vi "Multistate LED Example LV2012.vi"() -> ()   [LabVIEW 2012]
panel:
  in  "stop":bool
  out "Color Box":u32(colorbox)
  in  "Enum":T1(ring)
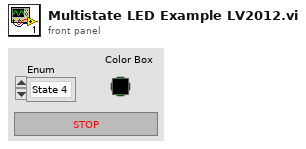
[diagram p1: front panel]
types:
  T1 = enum16{"State 4", "State 3", "State 2", "State 1", "State 0"}
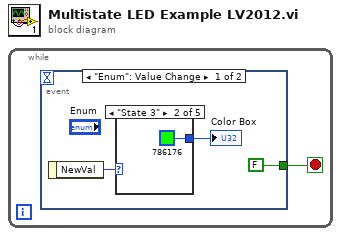
[diagram p0: block diagram]
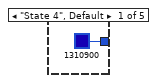
[diagram p2: hidden frame]
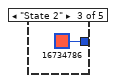
[diagram p3: hidden frame]
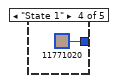
[diagram p4: hidden frame]
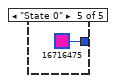
[diagram p5: hidden frame]
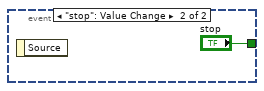
[diagram p6: hidden frame]
diagram:
  n1 = while {
    stop <- w1 stop-if-true
    n2 = event shown="[0] \"Enum\": Value Change" {
      selector: _ -> [_ _]
      dyn-events: _ -> [_ _]
      timeout: _ -> [_ _]
      tunnel: [FALSE ("stop") "stop"] -> w1
      event "Enum": Value Change {
        n3 = event-data() -> ("NewVal"=w3:T1)  [unwired: 1 in]
        n4 = case shown="\"State 3\"" w3 {
          tunnel: [u32 1310900 u32 786176 u32 16734786 u32 11771020 u32 16716475] -> w4
          frame "State 4", Default {
          }
          frame "State 3" {
          }
          frame "State 2" {
          }
          frame "State 1" {
          }
          frame "State 0" {
          }
        }
        "Color Box" <- w4
      }
      event "stop": Value Change {
        n5 = event-data() -> ()  [unwired: 1 in, 1 out]
      }
    }
  }
